vi "Filter Triggered.vi"(8 "error in (no error)":errorcluster, 10 "Assert Message":T1, 11 "Base Filter in":refnum<class "Base Filter.lvclass">) -> (0 "error out":errorcluster, 2 "Filtered":bool)   [LabVIEW 2016, in "Assert API Components.lvlib" / "Base Filter.lvclass"]
uses:
  Base Filter.lvclass
  Message Data.ctl
  Failure Actions.ctl
  VI References.ctl
  Base Filter.lvclass/Base Filter.ctl
  Assert API Components.lvlib
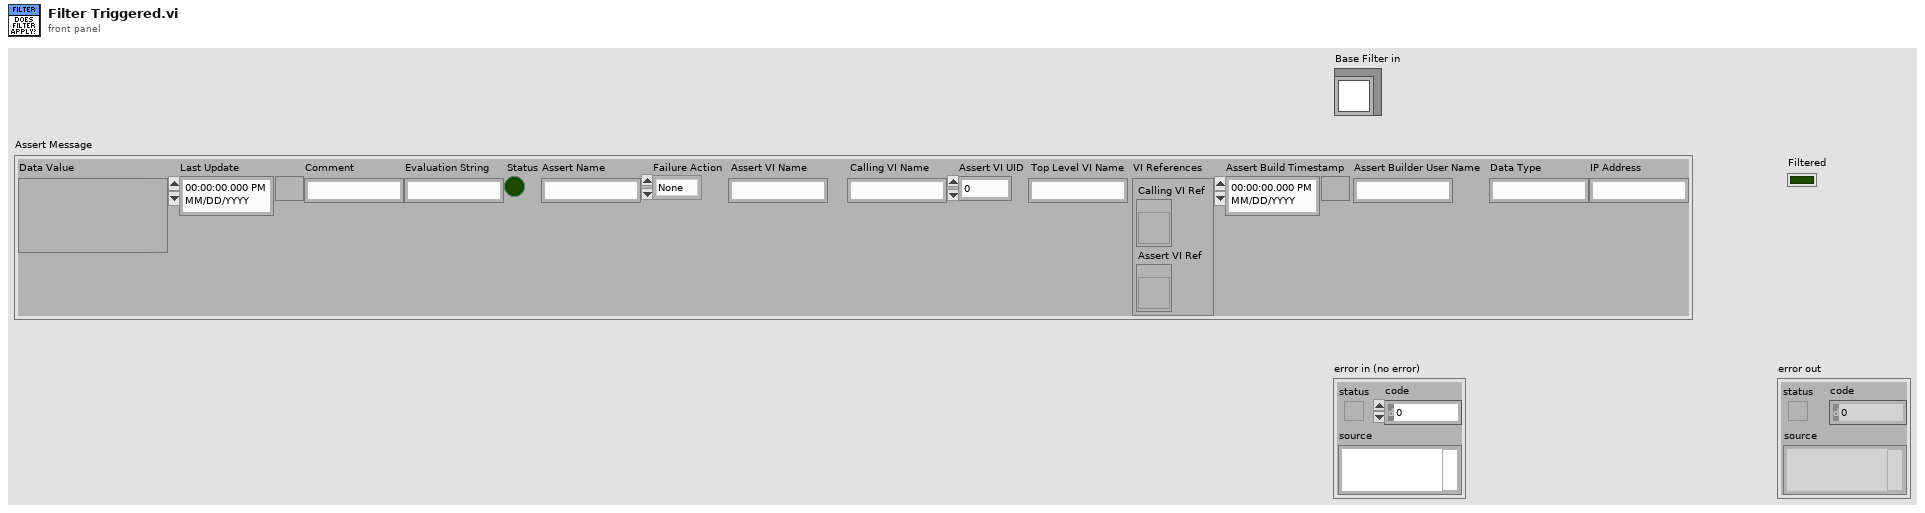
[diagram p1: front panel]
types:
  T1 = typedef "Assert API Components.lvlib/Message Data.ctl" = cluster{"Data Value":variant, "Last Update":timestamp, "Comment":string, "Evaluation String":string, "Status":bool, "Assert Name":string, "Failure Action":T2, "Assert VI Name":string, "Calling VI Name":string, "Assert VI UID":i32, "Top Level VI Name":string, "VI References":T3, "Assert Build Timestamp":timestamp, "Assert Builder User Name":string, "Data Type":string, "IP Address":string}
  T2 = typedef "Assert API Components.lvlib/Failure Actions.ctl" = enum16{"None", "Log To File", "Pause Execution", "Abort Execution"}
  T3 = typedef "Assert API Components.lvlib/VI References.ctl" = cluster{"Calling VI Ref":refnum<vi>, "Assert VI Ref":refnum<vi>}
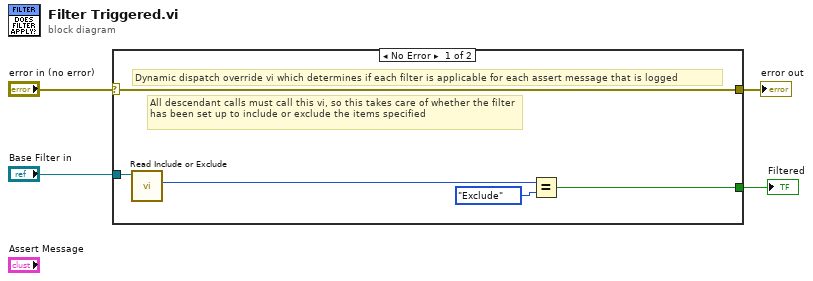
[diagram p0: block diagram]
diagram:
  n1 = case shown="No Error" "error in (no error)" {
    selector: "error in (no error)" -> [w9 w10]
    tunnel: [w9 w10] -> w3
    tunnel: "Base Filter in" -> [w8 _]
    tunnel: [w5 _] -> w1
    frame No Error {
      # "All descendant calls must call this vi, so this takes care of whether the filter has been set up to include or exclude the items specified"
      # "Dynamic dispatch override vi which determines if each filter is applicable for each assert message that is logged"
      n2 = call "Read Include or Exclude.vi"("Base Filter in"=w8) -> ("Include or Exclude"=w7:enum16{"Include", "Exclude"})  [unwired: 10 in]
      n3 = Equal?(x=w7, y=enum16{"Include", "Exclude"}."Exclude") -> (x = y?=w5:bool)
    }
    frame Error {
    }
  }
  "error out" <- w3
  "Filtered" <- w1
